vi "Esercitazione 6 - Array contenitore e contenuto.vi"() -> ()   [LabVIEW 2018]
panel:
  out "Boolean":bool
  in  "Array contenuto":dbl[](array[numeric])
  in  "Array contenitore":dbl[](array[numeric])
  # "array contenuto"
  # "array contenitore"
  # "verificare che ogni elem\ndel 2o array sia presente\nnel 1o array"
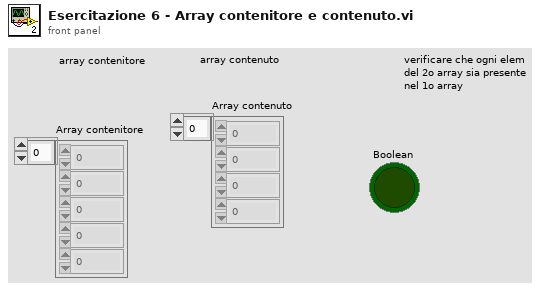
[diagram p1: front panel]
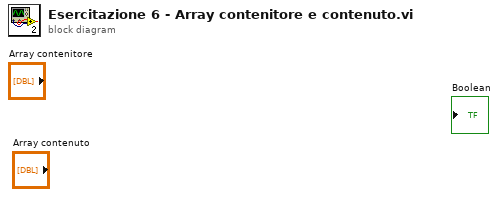
[diagram p0: block diagram]
diagram:
